vi "Shutdown S3DK.vi"(8 "error in (no error)":errorcluster, 11 "Hardware Resources in":T1={"State"=enum."Idle S3DK", "Settings"="", "Online"=FALSE, "S3DK"={"Signals"={"Phasor"=[], "Analog"=[], "Digital"=[]}}, "CSV"={"CSV Path"=path "", "Index"=0, "Parcel Length"=0, "EOF?"=FALSE}}) -> (0 "error out":errorcluster)   [LabVIEW 2017, in "Acquisition.lvlib"]
doc: "Stops the acquisition."
uses:
  Acquisition.lvlib
  Acquisition Settings.ctl
  Acquisition State.ctl
  <vilib>/S3DK/PMU Recorder Light/PMU Recorder Light.lvlib
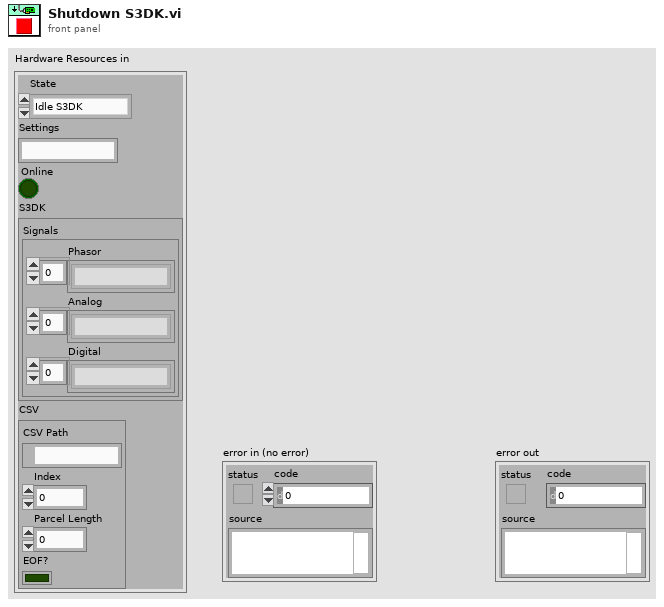
[diagram p1: front panel]
types:
  T1 = typedef "Acquisition.lvlib/Acquisition Settings.ctl" = cluster{"State":T2, "Settings":string, "Online":bool, "S3DK":cluster{"Signals":cluster{"Phasor":string[], "Analog":string[], "Digital":string[]}}, "CSV":cluster{"CSV Path":path, "Index":i32, "Parcel Length":i32, "EOF?":bool}}
  T2 = typedef "Acquisition.lvlib/Acquisition State.ctl" = enum16{"Idle", "Idle S3DK", "Acquiring S3DK", "Idle CSV", "Acquiring CSV"}
  T3 = enum16{"Run", "Startup", "Get Status", "Pause", "Continue", "Shutdown", "Abort", "Open Panel", "Close Panel"}
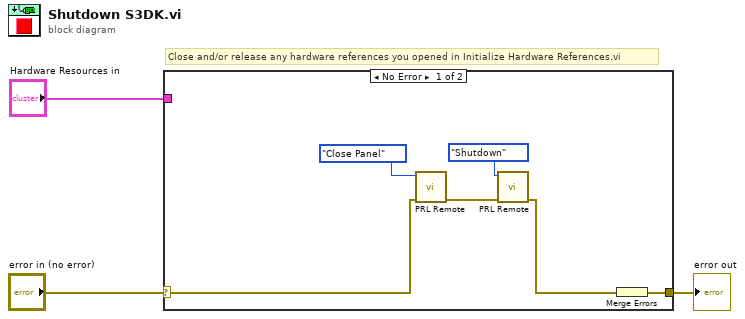
[diagram p0: block diagram]
diagram:
  # "Close and/or release any hardware references you opened in Initialize Hardware References.vi"
  n1 = case shown="No Error" "error in (no error)" {
    selector: "error in (no error)" -> [w4 w10]
    tunnel: [w9 w10] -> w2
    tunnel: "Hardware Resources in" -> [_ _]
    frame No Error {
      n2 = call <vilib>:"PRL Remote.vi"("error in (no error)"=w4, "Action"=T3."Close Panel") -> ("error out"=w6:errorcluster)  [unwired: 4 in, 5 out]
      n3 = call <vilib>:"PRL Remote.vi"("error in (no error)"=w6, "Action"=T3."Shutdown") -> ("error out"=w7:errorcluster)  [unwired: 4 in, 5 out]
      n4 = Merge Errors(w7) -> (w9:errorcluster)
    }
    frame Error {
    }
  }
  "error out" <- w2
